vi "Show_Process_Steps.vi"(8 "error in (no error)":errorcluster, 10 "ProcessSettingIn":T8[](array[typedef]), 11 "ProcessSteps":refnum<vi>) -> (0 "error out":errorcluster)   [LabVIEW 2019]
uses:
  Controls/MaskParam_Type.ctl
  Controls/BinaryMonoParam_Type.ctl
  Controls/Process_Setting.ctl
  Controls/OperatorsParam_Type.ctl
  Controls/GrayMorphologyParam_Type.ctl
  Controls/FiltersParam_Type.ctl
  Controls/LookupTableParam.ctl
  Controls/ParticleFilterParam_Type.ctl
  Controls/ExtractPlanParam_Type.ctl
  Ctrl/VisionProcessName.ctl
panel:
  in  "ExtractPlanParam":T1={"Color Plane"=enum."Blue"}
  in  "ParticleFilterParam":T2={"Selection Values"=[{"Measurement Parameter"=16, "Range Lower Value"=0.0, "Range Upper Value"=0.0, "Range"=FALSE, "Measurement Type"=FALSE}], "Keep/Remove Particles (F)"=FALSE, "Reject Border? (F)"=FALSE, "Fill Holes? (F)"=FALSE, "Connectivity 4/8 (8)"=FALSE} {"Selection Values"."Measurement Parameter" items=["Center of Mass X", "Center of Mass Y", "First Pixel X", "First Pixel Y", "Bounding Rect Left", "Bounding Rect Top", "Bounding Rect Right", "Bounding Rect Bottom", "Max Feret Diameter Start X", "Max Feret Diameter Start Y", "Max Feret Diameter End X", "Max Feret Diameter End Y", "Max Horiz. Segment Length Left", "Max Horiz. Segment Length Right", "Max Horiz. Segment Length Row", "-", "Bounding Rect Width", "Bounding Rect Height", "Bounding Rect Diagonal", "Perimeter", "Convex Hull Perimeter", "Holes' Perimeter", "Max Feret Diameter", "Equivalent Ellipse Major Axis", "Equivalent Ellipse Minor Axis", "Equivalent Ellipse Minor Axis (Feret)", "Equivalent Rect Long Side", "Equivalent Rect Short Side", "Equivalent Rect Diagonal", "Equivalent Rect Short Side (Feret)", "Average Horiz. Segment Length", "Average Vert. Segment Length", "Hydraulic Radius", "Waddel Disk Diameter", "-", "Area", "Holes' Area", "Particle & Holes' Area", "Convex Hull Area", "Image Area", "-", "Number of Holes", "Number of Horiz. Segments", "Number of Vert. Segments", "-", "Orientation", "Max Feret Diameter Orientation", "-", "% Area/Image Area", "% Area/(Particle & Holes' Area)", "Ratio of Equivalent Ellipse Axes", "Ratio of Equivalent Rect Sides", "-", "Elongation Factor", "Compactness Factor", "Heywood Circularity Factor", "Type Factor", "-", "Sum X", "Sum Y", "Sum XX", "Sum XY", "Sum YY", "Sum XXX", "Sum XXY", "Sum XYY", "Sum YYY", "-", "Moment of Inertia XX", "Moment of Inertia XY", "Moment of Inertia YY", "Moment of Inertia XXX", "Moment of Inertia XXY", "Moment of Inertia XYY", "Moment of Inertia YYY", "Norm. Moment of Inertia XX", "Norm. Moment of Inertia XY", "Norm. Moment of Inertia YY", "Norm. Moment of Inertia XXX", "Norm. Moment of Inertia XXY", "Norm. Moment of Inertia XYY", "Norm. Moment of Inertia YYY", "Hu Moment 1", "Hu Moment 2", "Hu Moment 3", "Hu Moment 4", "Hu Moment 5", "Hu Moment 6", "Hu Moment 7"]; "Selection Values"."Range Lower Value" format="%.2f"; "Selection Values"."Range Upper Value" format="%.2f"}
  in  "LookupTableParam":T4
  in  "FiltersParam":T5={"Kernel"=[[1.0, 1.0, 1.0], [1.0, 1.0, 1.0], [1.0, 1.0, 1.0]], "Kernel Size"=0, "Filter Size X"=0, "Filter Size Y"=0, "Tolerance %"=0, "Divider"=0.0, "FilterFunction"=enum."Smoothing - Low Pass", "Sigma"=0.0, "LThres"=0.0, "HThresh"=0.0, "Windows Size"=0} {"Kernel Size" min=3 max=7 step=2}
  in  "GrayMorphologyParam":T6={"Operation"=enum."Gradient in", "Structuring Element"=[[1, 1, 1], [1, 1, 1], [1, 1, 1]], "Square/Hexa (Square)"=TRUE, "Number of iterations"=1}
  in  "OperatorsParam":T7
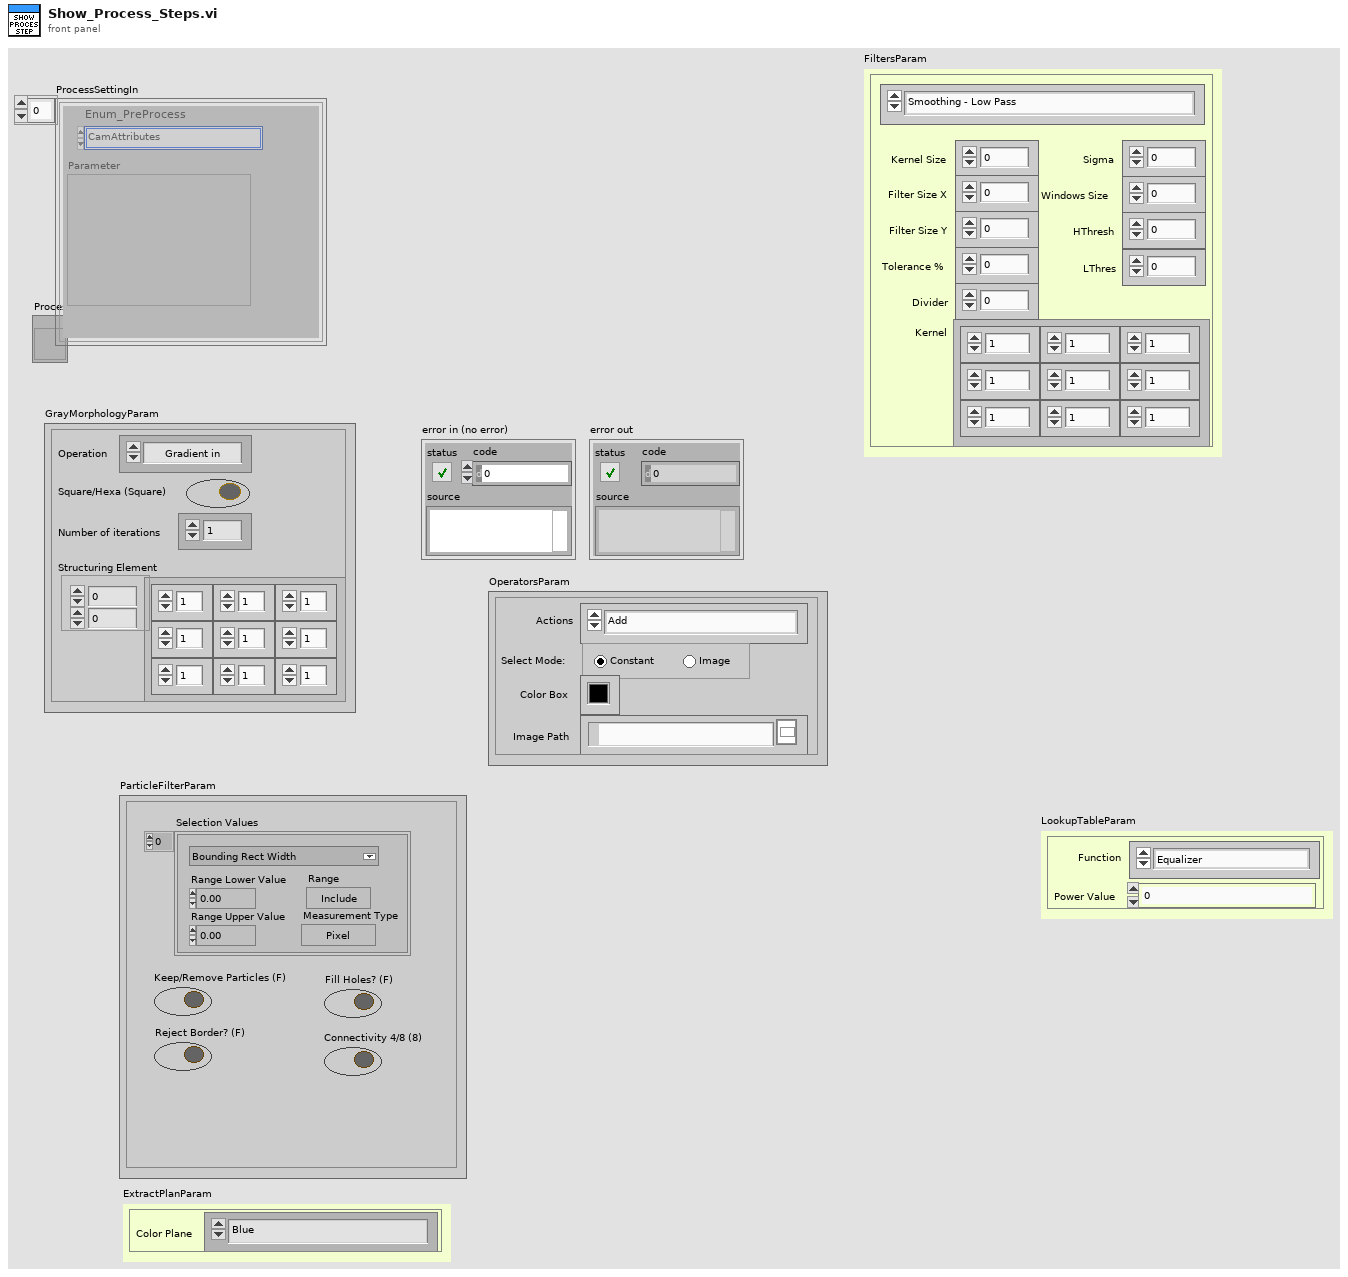
[diagram p1: front panel]
types:
  T1 = typedef "ExtractPlanParam_Type.ctl" = cluster{"Color Plane":enum16{"Red", "Green", "Blue", "Hue", "Saturation", "Luminance", "Value", "Intensity"}}
  T2 = typedef "ParticleFilterParam_Type.ctl" = cluster{"Selection Values":cluster{"Measurement Parameter":T3, "Range Lower Value":dbl, "Range Upper Value":dbl, "Range":bool, "Measurement Type":bool}[], "Keep/Remove Particles (F)":bool, "Reject Border? (F)":bool, "Fill Holes? (F)":bool, "Connectivity 4/8 (8)":bool}
  T3 = typedef "Particle Parameters" = i32
  T4 = typedef "LookupTableParam.ctl" = cluster{"Function":enum16{"Equalizer", "Reverse", "Logarithmic", "Exponential", "Square", "Square Root", "Power X", "Power 1/X"}, "Power Value":sgl}
  T5 = typedef "FiltersParam_Type.ctl" = cluster{"Kernel":sgl[][], "Kernel Size":i32, "Filter Size X":i32, "Filter Size Y":i32, "Tolerance %":i32, "Divider":sgl, "FilterFunction":enum16{"Smoothing - Low Pass", "Smoothing - Local Average", "Smoothing - Guassian", "Smoothing - Median", "------------------------------------", "Edge Detection - Laplacian", "Edge Detection - Diff", "Edge Detection - Prewitt", "Edge Detection - Sobel", "Edge Detection - Roberts", "Edge Detection - Canny", "Edge Detection - Gradient", "Edge Detection - Sigma", "----------------------------------------", "Convolution - Highlight Details", "Convolution - Custom"}, "Sigma":sgl, "LThres":sgl, "HThresh":sgl, "Windows Size":i32}
  T6 = typedef "GrayMorphologyParam_Type.ctl" = cluster{"Operation":enum32{"AutoM", "Close", "Dilate", "Erode", "Gradient", "Gradient in", "Gradient out", "HitMiss", "Open", "PClose", "POpen", "Thick", "Thin"}, "Structuring Element":i32[][], "Square/Hexa (Square)":bool, "Number of iterations":i32}
  T7 = typedef "OperatorsParam_Type.ctl" = cluster{"Actions":enum16{"Add", "Subtract", "Multiply", "Divide", "Multiply Divide", "Modulo", "Absolutio Difference", "---------------------------------", "And", "Not And", "Or", "Not Or", "Exclusive Or", "Not Exclusive Or", "Logical Difference", "----------------------------------", "Mask"}, "Select Mode:":enum32{"Constant", "Image"}, "Color Box":u32, "Image Path":path}
  T8 = typedef "Process_Setting.ctl" = cluster{"Enum_PreProcess":T9, "Parameter":string}
  T9 = typedef "VisionProcessName.ctl" = enum16{"*CamParameter*", "CamAttributes", "*Preprocess*", "CG_Brightness", "C_Plane Extraction", "C_Threshold", "G_Lookup Table", "G_Threshold"}
  T10 = typedef "MaskParam_Type.ctl" = cluster{"Function":enum16{"Inside", "Outside"}, "ROI List":i32, "ROI":cluster{"Global Rectangle":i32[], "Contours":cluster{"Contour Type":u32, "ROI Type":u32, "Points":i32[]}[]}[], "Creat ROI":bool, "Delete ROI":bool, "Enabled/Disabled":bool, "Color Box":u32, "Last Mouse Position":cluster{"X":i32, "Y":i32}}
  T11 = typedef "BinaryMonoParam_Type.ctl" = cluster{"Look For":enum16{"Bright Objects", "Dark Objects", "Gray Objects"}, "Threshold":cluster{dbl, dbl}}
  T12 = typedef "Process_Type.ctl" = enum16{"None", "ExtractPlane", "BinaryMono", "Operators", "GrayMorphology", "Filters", "Lookup Table", "Particle Filter", "Mask"}
  T13 = enum16{"Red", "Green", "Blue", "Hue", "Saturation", "Luminance", "Value", "Intensity"}
  T14 = enum16{"Add", "Subtract", "Multiply", "Divide", "Multiply Divide", "Modulo", "Absolutio Difference", "---------------------------------", "And", "Not And", "Or", "Not Or", "Exclusive Or", "Not Exclusive Or", "Logical Difference", "----------------------------------", "Mask"}
  T15 = enum32{"AutoM", "Close", "Dilate", "Erode", "Gradient", "Gradient in", "Gradient out", "HitMiss", "Open", "PClose", "POpen", "Thick", "Thin"}
  T16 = enum16{"Smoothing - Low Pass", "Smoothing - Local Average", "Smoothing - Guassian", "Smoothing - Median", "------------------------------------", "Edge Detection - Laplacian", "Edge Detection - Diff", "Edge Detection - Prewitt", "Edge Detection - Sobel", "Edge Detection - Roberts", "Edge Detection - Canny", "Edge Detection - Gradient", "Edge Detection - Sigma", "----------------------------------------", "Convolution - Highlight Details", "Convolution - Custom"}
  T17 = enum16{"Equalizer", "Reverse", "Logarithmic", "Exponential", "Square", "Square Root", "Power X", "Power 1/X"}
  T18 = cluster{"Measurement Parameter":T3, "Range Lower Value":dbl, "Range Upper Value":dbl, "Range":bool, "Measurement Type":bool}[]
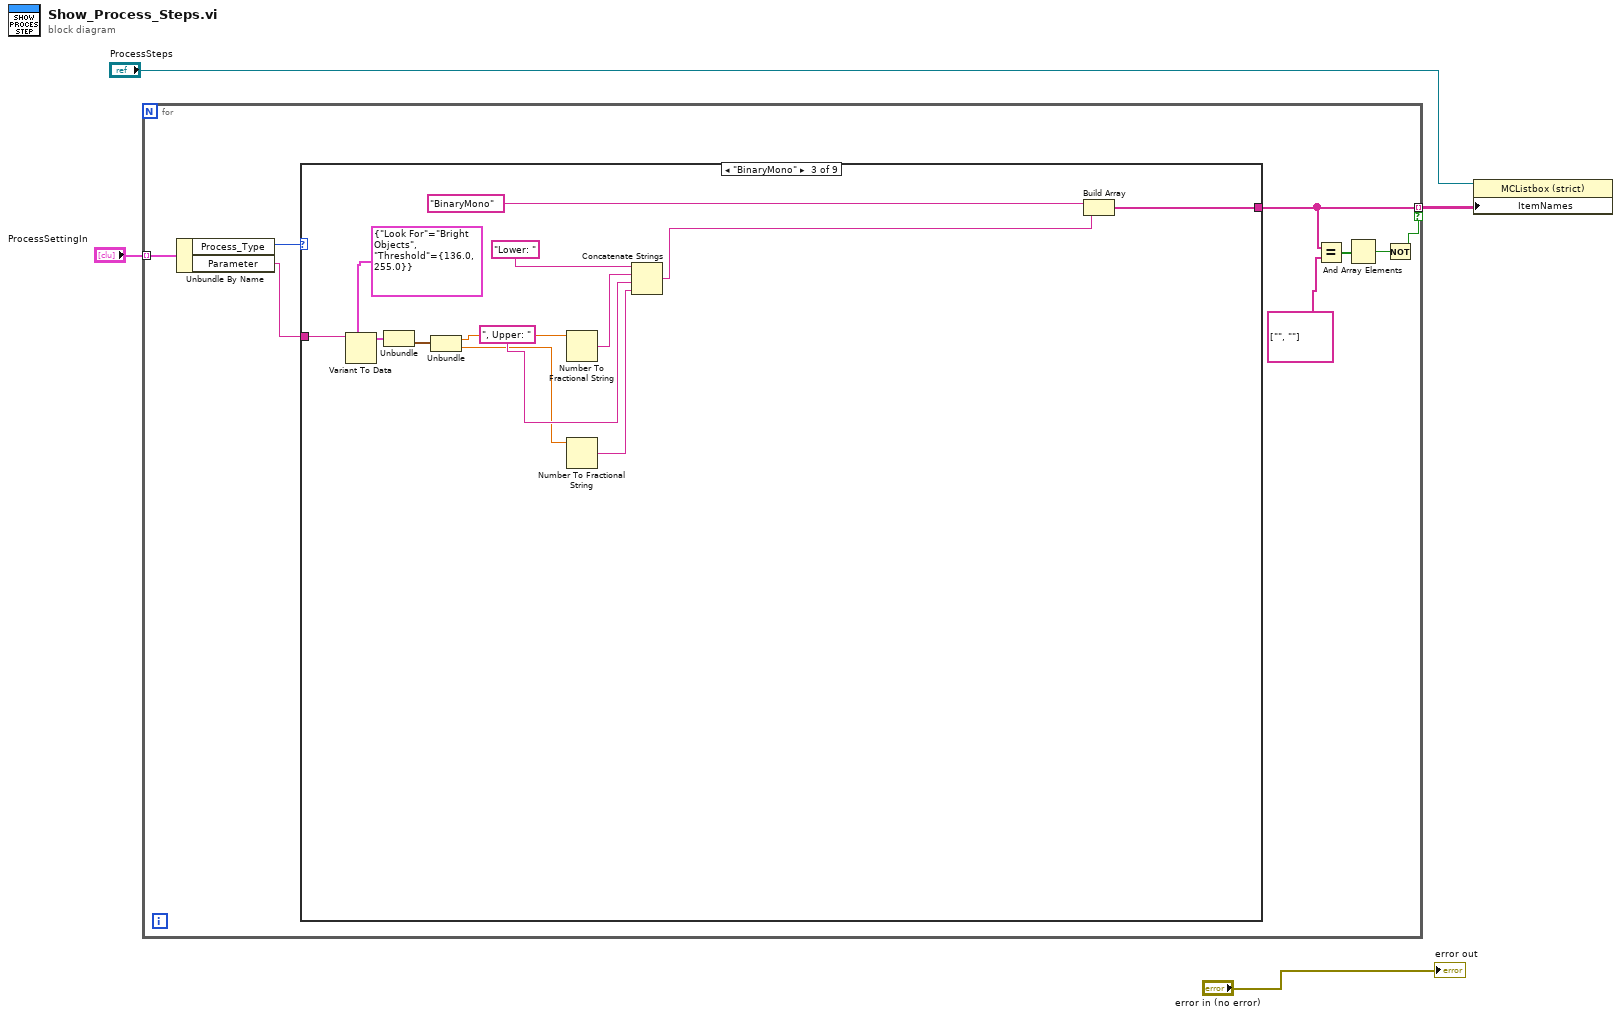
[diagram p0: block diagram]
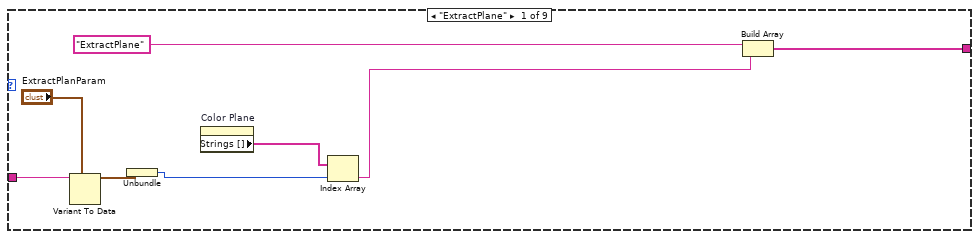
[diagram p2: hidden frame]
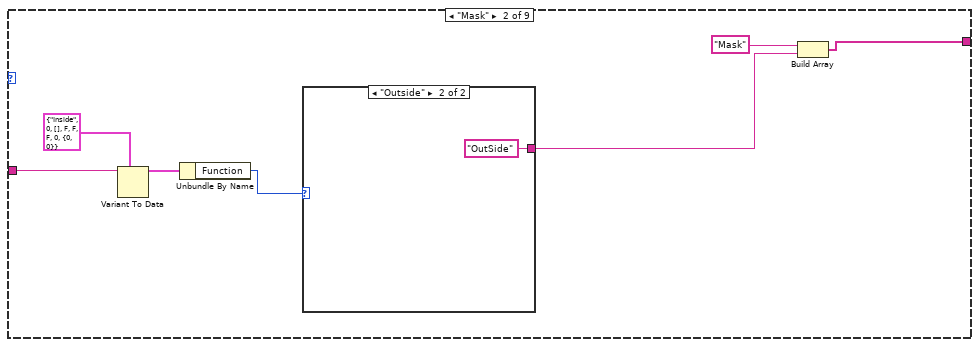
[diagram p3: hidden frame]
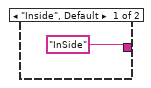
[diagram p4: hidden frame]
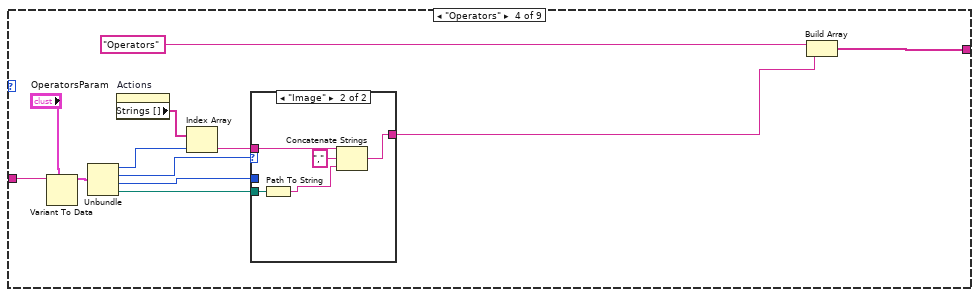
[diagram p5: hidden frame]
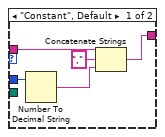
[diagram p6: hidden frame]
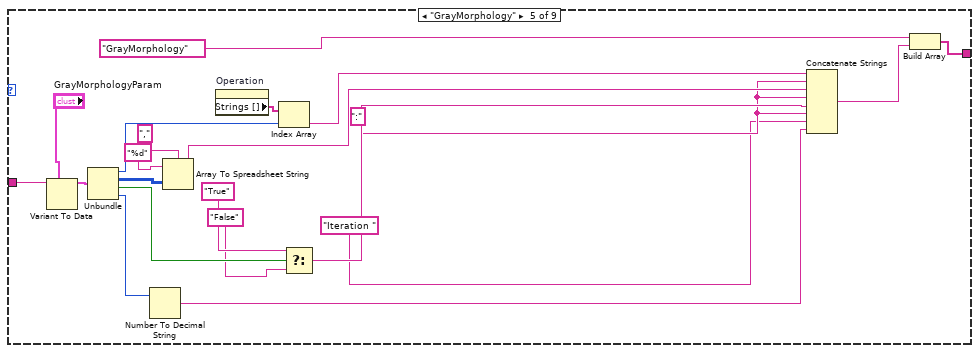
[diagram p7: hidden frame]
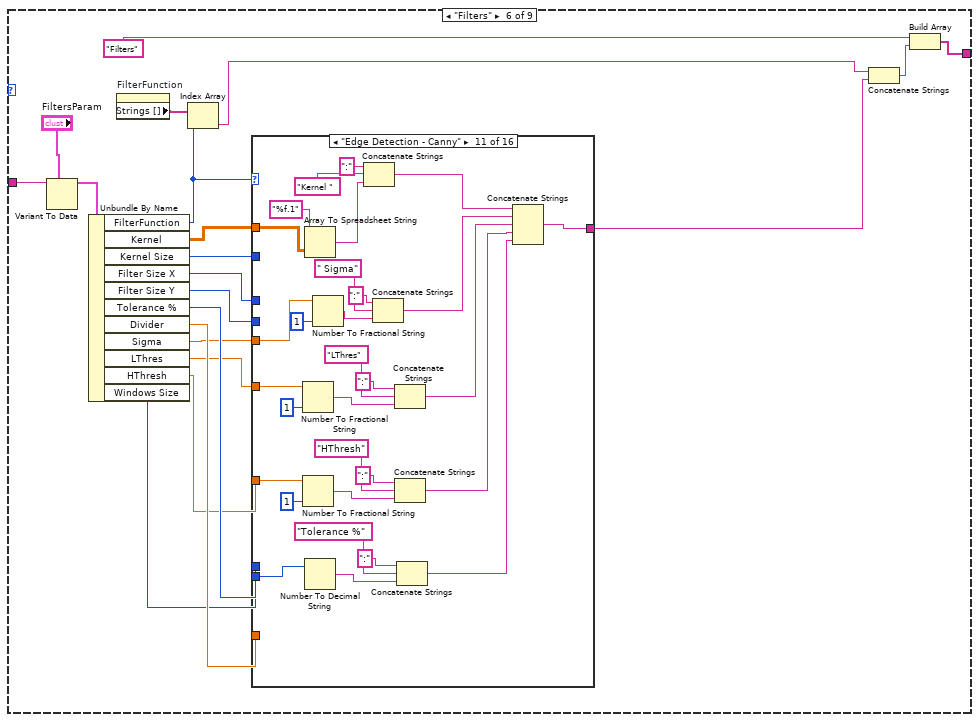
[diagram p8: hidden frame]
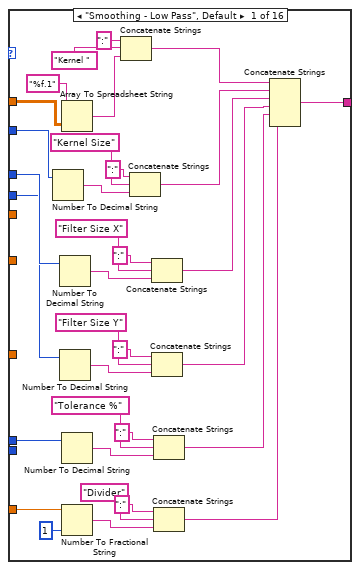
[diagram p9: hidden frame]
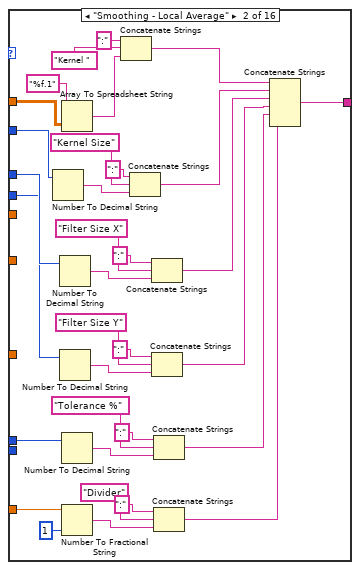
[diagram p10: hidden frame]
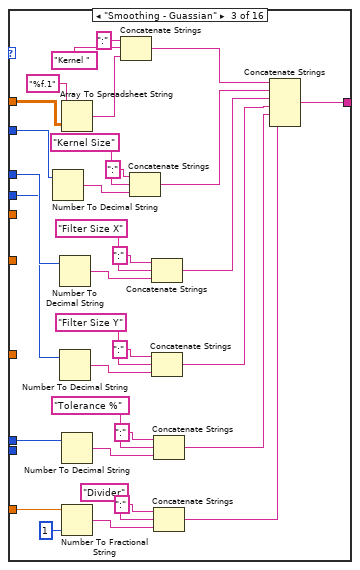
[diagram p11: hidden frame]
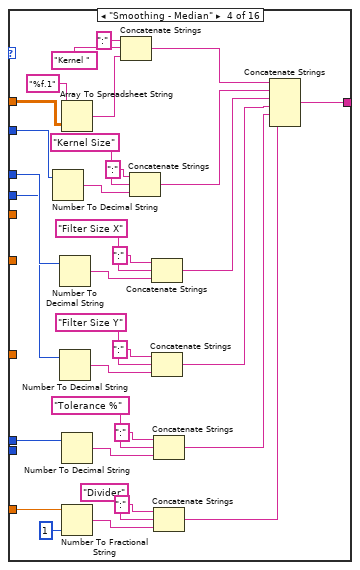
[diagram p12: hidden frame]
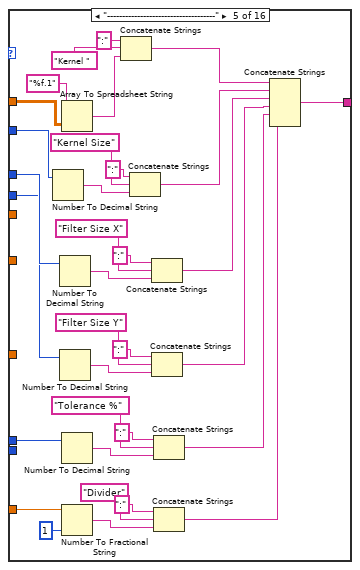
[diagram p13: hidden frame]
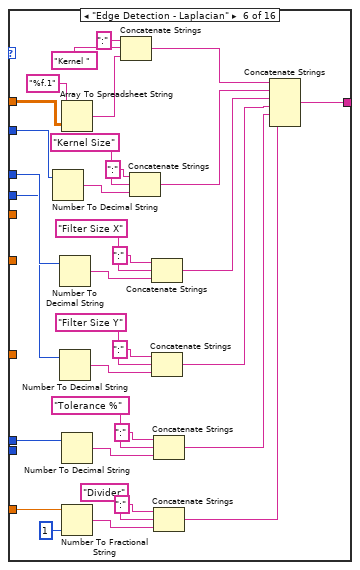
[diagram p14: hidden frame]
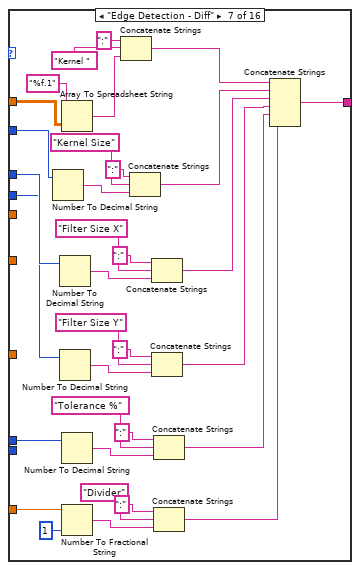
[diagram p15: hidden frame]
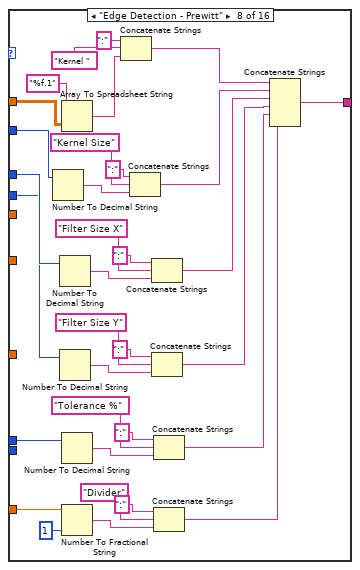
[diagram p16: hidden frame]
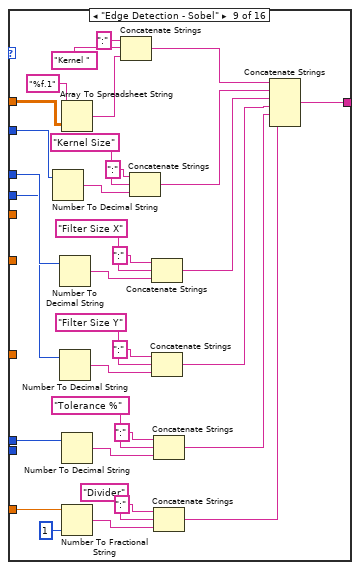
[diagram p17: hidden frame]
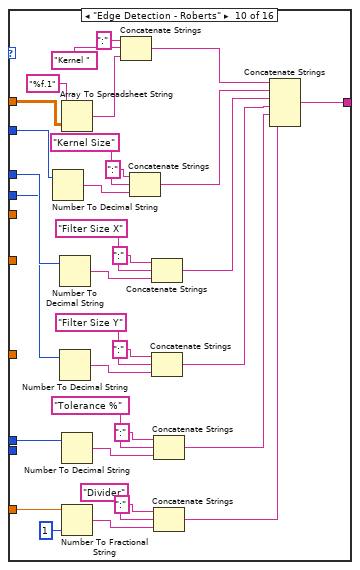
[diagram p18: hidden frame]
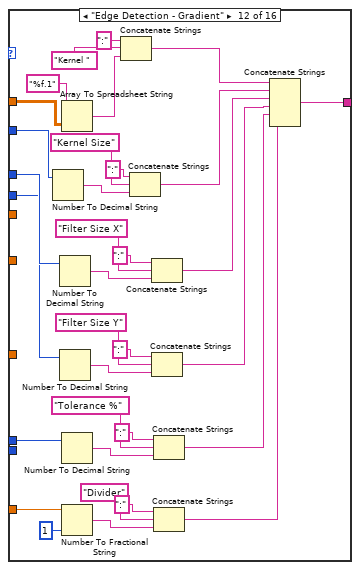
[diagram p19: hidden frame]
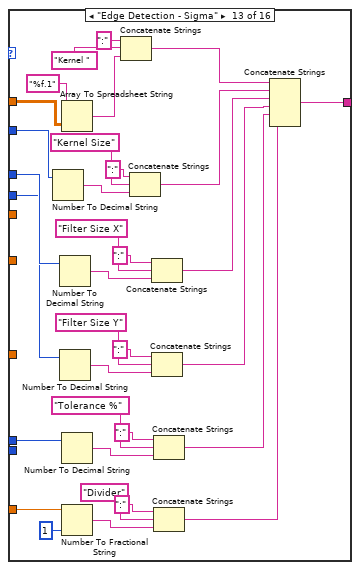
[diagram p20: hidden frame]
diagram:
  n1 = for {
    tunnel: "ProcessSettingIn" -> [w12] mode=indexing
    tunnel: [w9] -> w2 mode=indexing if=w5
    n2 = Unbundle By Name(w12) -> ("Process_Type"=w11:T12, "Parameter"=w10:string)
    n3 = case shown="\"BinaryMono\"" w11 {
      tunnel: w10 -> [w20 w25 w42 w54 w85 w105 w640 w696 _]
      tunnel: [w17 w27 w40 w43 w67 w103 w631 w693 _] -> w9
      frame "ExtractPlane" {
        n4 = Variant To Data(type="ExtractPlanParam", Variant=w20) -> (data=w16:T1)  [unwired: 1 in, 1 out]
        n5 = Unbundle(w16) -> ("Color Plane"=w15:T13)
        n6 = property on="Color Plane" class="Enum (strict)"() -> ("Strings []"=w14:string[])  [unwired: 2 in, 2 out]
        n7 = Index Array(array=w14, index=w15) -> (element=w18:string)
        n8 = Build Array("ExtractPlane", w18) -> (w17:string[])
      }
      frame "Mask" {
        n9 = Variant To Data(type=T10 {"Function"=enum."Inside", "ROI List"=0, "ROI"=[], "Creat ROI"=FALSE, "Delete ROI"=FALSE, "Enabled/Disabled"=FALSE, "Color Box"=0, "Last Mouse Position"={"X"=0, "Y"=0}} ("MaskParam"), Variant=w25) -> (data=w23:T10)  [unwired: 1 in, 1 out]
        n10 = Unbundle By Name(w23) -> ("Function"=w22:enum16{"Inside", "Outside"})
        n11 = case shown="\"Outside\"" w22 {
          tunnel: ["InSide" "OutSide"] -> w21
          frame "Inside", Default {
          }
          frame "Outside" {
          }
        }
        n12 = Build Array("Mask", w21) -> (w27:string[])
      }
      frame "BinaryMono" {
        n13 = Variant To Data(type=T11 {"Look For"=enum."Bright Objects", "Threshold"={136.0, 255.0}} ("BinaryMonoParam"), Variant=w42) -> (data=w34:T11)  [unwired: 1 in, 1 out]
        n14 = Unbundle(w34) -> ("Threshold"=w33:cluster{dbl, dbl})  [unwired: 1 out]
        n15 = Unbundle(w33) -> (w31:dbl, w32:dbl)
        n16 = Number To Fractional String(number=w31) -> (F-format string=w37:string)  [unwired: 3 in]
        n17 = Number To Fractional String(number=w32) -> (F-format string=w35:string)  [unwired: 3 in]
        n18 = Concatenate Strings("Lower: " ("string"), w37, ", Upper: " ("string"), w35) -> (w38:string)
        n19 = Build Array("BinaryMono", w38) -> (w40:string[])
      }
      frame "Operators" {
        n20 = Variant To Data(type="OperatorsParam", Variant=w54) -> (data=w52:T7)  [unwired: 1 in, 1 out]
        n21 = Unbundle(w52) -> ("Actions"=w49:T14, "Select Mode:"=w51:enum32{"Constant", "Image"}, "Color Box"=w47:u32, "Image Path"=w44:path)
        n22 = property on="Actions" class="Enum (strict)"() -> ("Strings []"=w50:string[])  [unwired: 2 in, 2 out]
        n23 = Index Array(array=w50, index=w49) -> (element=w48:string)
        n24 = case shown="\"Image\"" w51 {
          tunnel: w48 -> [w58 w64]
          tunnel: w47 -> [w59 _]
          tunnel: [w55 w62] -> w45
          tunnel: w44 -> [_ w61]
          frame "Constant", Default {
            n25 = Number To Decimal String(number=w59) -> (decimal integer string=w56:string)  [unwired: 1 in]
            n26 = Concatenate Strings(w58, "," ("string"), w56) -> (w55:string)
          }
          frame "Image" {
            n27 = Path To String(path=w61) -> (string=w60:string)
            n28 = Concatenate Strings(w64, "," ("string"), w60) -> (w62:string)
          }
        }
        n29 = Build Array("Operators", w45) -> (w43:string[])
      }
      frame "GrayMorphology" {
        w71 = ":" ("element")
        n30 = Variant To Data(type="GrayMorphologyParam", Variant=w85) -> (data=w84:T6)  [unwired: 1 in, 1 out]
        n31 = Unbundle(w84) -> ("Operation"=w81:T15, "Structuring Element"=w80:i32[][], "Square/Hexa (Square)"=w75:bool, "Number of iterations"=w70:i32)
        n32 = Number To Decimal String(number=w70) -> (decimal integer string=w66:string)  [unwired: 1 in]
        n33 = Array To Spreadsheet String(delimiter (Tab)=",", array=w80, 3:"%d" ("format string")) -> (spreadsheet string=w76:string)
        n34 = property on="Operation" class="Enum (strict)"() -> ("Strings []"=w82:string[])  [unwired: 2 in, 2 out]
        n35 = Index Array(array=w82, index=w81) -> (element=w77:string)
        n36 = Select(t="True" ("delimiter (Tab)"), s=w75, f="False" ("delimiter (Tab)")) -> (s? t:f=w72:string)
        n37 = Concatenate Strings(w77, w71, w76, w71, w72, w71, "Iteration " ("string"), w66) -> (w69:string)
        n38 = Build Array("GrayMorphology", w69) -> (w67:string[])
      }
      frame "Filters" {
        n39 = Variant To Data(type="FiltersParam", Variant=w105) -> (data=w100:T5)  [unwired: 1 in, 1 out]
        n40 = Unbundle By Name(w100) -> ("FilterFunction"=w99:T16, "Kernel"=w98:sgl[][], "Kernel Size"=w96:i32, "Filter Size X"=w95:i32, "Filter Size Y"=w94:i32, "Tolerance %"=w93:i32, "Divider"=w92:sgl, "Sigma"=w89:sgl, "LThres"=w88:sgl, "HThresh"=w87:sgl, "Windows Size"=w86:i32)
        n41 = property on="FilterFunction" class="Enum (strict)"() -> ("Strings []"=w101:string[])  [unwired: 2 in, 2 out]
        n42 = Index Array(array=w101, index=w99) -> (element=w97:string)
        n43 = case shown="\"Edge Detection - Canny\"" w99 {
          tunnel: w98 -> [w136 w169 w202 w235 w268 w301 w334 w367 w400 w433 w463 w496 w529 w562 w595 w628]
          tunnel: w96 -> [w133 w166 w199 w232 w265 w298 w331 w364 w397 w430 _ w493 w526 w559 w592 w625]
          tunnel: w95 -> [w126 w159 w192 w225 w258 w291 w324 w357 w390 w423 _ w486 w519 w552 w585 w618]
          tunnel: w94 -> [w122 w155 w188 w221 w254 w287 w320 w353 w386 w419 _ w482 w515 w548 w581 w614]
          tunnel: w93 -> [w118 w151 w184 w217 w250 w283 w316 w349 w382 w415 _ w478 w511 w544 w577 w610]
          tunnel: w92 -> [w113 w146 w179 w212 w245 w278 w311 w344 w377 w410 _ w473 w506 w539 w572 w605]
          tunnel: [w106 w139 w172 w205 w238 w271 w304 w337 w370 w403 w443 w466 w499 w532 w565 w598] -> w91
          tunnel: w89 -> [_ _ _ _ _ _ _ _ _ _ w442 _ _ _ _ _]
          tunnel: w88 -> [_ _ _ _ _ _ _ _ _ _ w440 _ _ _ _ _]
          tunnel: w87 -> [_ _ _ _ _ _ _ _ _ _ w438 _ _ _ _ _]
          tunnel: w86 -> [_ _ _ _ _ _ _ _ _ _ w436 _ _ _ _ _]
          frame "Smoothing - Low Pass", Default {
            n44 = Number To Decimal String(number=w133) -> (decimal integer string=w131:string)  [unwired: 1 in]
            n45 = Number To Decimal String(number=w126) -> (decimal integer string=w128:string)  [unwired: 1 in]
            n46 = Number To Decimal String(number=w122) -> (decimal integer string=w124:string)  [unwired: 1 in]
            n47 = Array To Spreadsheet String(array=w136, 3:"%f.1" ("format string")) -> (spreadsheet string=w134:string)  [unwired: 1 in]
            n48 = Number To Decimal String(number=w118) -> (decimal integer string=w120:string)  [unwired: 1 in]
            n49 = Number To Fractional String(number=w113, precision (6)=i16 1) -> (F-format string=w116:string)  [unwired: 2 in]
            n50 = Concatenate Strings(":" ("string"), "Kernel " ("string"), w134) -> (w112:string)
            n51 = Concatenate Strings(":" ("string"), "Kernel Size" ("string"), w131) -> (w111:string)
            n52 = Concatenate Strings(":" ("string"), "Filter Size X" ("string"), w128) -> (w110:string)
            n53 = Concatenate Strings(":" ("string"), "Filter Size Y" ("string"), w124) -> (w109:string)
            n54 = Concatenate Strings(":" ("string"), "Tolerance %" ("string"), w120) -> (w108:string)
            n55 = Concatenate Strings(":" ("string"), "Divider" ("string"), w116) -> (w107:string)
            n56 = Concatenate Strings(w112, w111, w110, w109, w108, w107) -> (w106:string)
          }
          frame "Smoothing - Local Average" {
            n57 = Number To Decimal String(number=w166) -> (decimal integer string=w164:string)  [unwired: 1 in]
            n58 = Number To Decimal String(number=w159) -> (decimal integer string=w161:string)  [unwired: 1 in]
            n59 = Number To Decimal String(number=w155) -> (decimal integer string=w157:string)  [unwired: 1 in]
            n60 = Array To Spreadsheet String(array=w169, 3:"%f.1" ("format string")) -> (spreadsheet string=w167:string)  [unwired: 1 in]
            n61 = Number To Decimal String(number=w151) -> (decimal integer string=w153:string)  [unwired: 1 in]
            n62 = Number To Fractional String(number=w146, precision (6)=i16 1) -> (F-format string=w149:string)  [unwired: 2 in]
            n63 = Concatenate Strings(":" ("string"), "Kernel " ("string"), w167) -> (w145:string)
            n64 = Concatenate Strings(":" ("string"), "Kernel Size" ("string"), w164) -> (w144:string)
            n65 = Concatenate Strings(":" ("string"), "Filter Size X" ("string"), w161) -> (w143:string)
            n66 = Concatenate Strings(":" ("string"), "Filter Size Y" ("string"), w157) -> (w142:string)
            n67 = Concatenate Strings(":" ("string"), "Tolerance %" ("string"), w153) -> (w141:string)
            n68 = Concatenate Strings(":" ("string"), "Divider" ("string"), w149) -> (w140:string)
            n69 = Concatenate Strings(w145, w144, w143, w142, w141, w140) -> (w139:string)
          }
          frame "Smoothing - Guassian" {
            n70 = Number To Decimal String(number=w199) -> (decimal integer string=w197:string)  [unwired: 1 in]
            n71 = Number To Decimal String(number=w192) -> (decimal integer string=w194:string)  [unwired: 1 in]
            n72 = Number To Decimal String(number=w188) -> (decimal integer string=w190:string)  [unwired: 1 in]
            n73 = Array To Spreadsheet String(array=w202, 3:"%f.1" ("format string")) -> (spreadsheet string=w200:string)  [unwired: 1 in]
            n74 = Number To Decimal String(number=w184) -> (decimal integer string=w186:string)  [unwired: 1 in]
            n75 = Number To Fractional String(number=w179, precision (6)=i16 1) -> (F-format string=w182:string)  [unwired: 2 in]
            n76 = Concatenate Strings(":" ("string"), "Kernel " ("string"), w200) -> (w178:string)
            n77 = Concatenate Strings(":" ("string"), "Kernel Size" ("string"), w197) -> (w177:string)
            n78 = Concatenate Strings(":" ("string"), "Filter Size X" ("string"), w194) -> (w176:string)
            n79 = Concatenate Strings(":" ("string"), "Filter Size Y" ("string"), w190) -> (w175:string)
            n80 = Concatenate Strings(":" ("string"), "Tolerance %" ("string"), w186) -> (w174:string)
            n81 = Concatenate Strings(":" ("string"), "Divider" ("string"), w182) -> (w173:string)
            n82 = Concatenate Strings(w178, w177, w176, w175, w174, w173) -> (w172:string)
          }
          frame "Smoothing - Median" {
            n83 = Number To Decimal String(number=w232) -> (decimal integer string=w230:string)  [unwired: 1 in]
            n84 = Number To Decimal String(number=w225) -> (decimal integer string=w227:string)  [unwired: 1 in]
            n85 = Number To Decimal String(number=w221) -> (decimal integer string=w223:string)  [unwired: 1 in]
            n86 = Array To Spreadsheet String(array=w235, 3:"%f.1" ("format string")) -> (spreadsheet string=w233:string)  [unwired: 1 in]
            n87 = Number To Decimal String(number=w217) -> (decimal integer string=w219:string)  [unwired: 1 in]
            n88 = Number To Fractional String(number=w212, precision (6)=i16 1) -> (F-format string=w215:string)  [unwired: 2 in]
            n89 = Concatenate Strings(":" ("string"), "Kernel " ("string"), w233) -> (w211:string)
            n90 = Concatenate Strings(":" ("string"), "Kernel Size" ("string"), w230) -> (w210:string)
            n91 = Concatenate Strings(":" ("string"), "Filter Size X" ("string"), w227) -> (w209:string)
            n92 = Concatenate Strings(":" ("string"), "Filter Size Y" ("string"), w223) -> (w208:string)
            n93 = Concatenate Strings(":" ("string"), "Tolerance %" ("string"), w219) -> (w207:string)
            n94 = Concatenate Strings(":" ("string"), "Divider" ("string"), w215) -> (w206:string)
            n95 = Concatenate Strings(w211, w210, w209, w208, w207, w206) -> (w205:string)
          }
          frame "------------------------------------" {
            n96 = Number To Decimal String(number=w265) -> (decimal integer string=w263:string)  [unwired: 1 in]
            n97 = Number To Decimal String(number=w258) -> (decimal integer string=w260:string)  [unwired: 1 in]
            n98 = Number To Decimal String(number=w254) -> (decimal integer string=w256:string)  [unwired: 1 in]
            n99 = Array To Spreadsheet String(array=w268, 3:"%f.1" ("format string")) -> (spreadsheet string=w266:string)  [unwired: 1 in]
            n100 = Number To Decimal String(number=w250) -> (decimal integer string=w252:string)  [unwired: 1 in]
            n101 = Number To Fractional String(number=w245, precision (6)=i16 1) -> (F-format string=w248:string)  [unwired: 2 in]
            n102 = Concatenate Strings(":" ("string"), "Kernel " ("string"), w266) -> (w244:string)
            n103 = Concatenate Strings(":" ("string"), "Kernel Size" ("string"), w263) -> (w243:string)
            n104 = Concatenate Strings(":" ("string"), "Filter Size X" ("string"), w260) -> (w242:string)
            n105 = Concatenate Strings(":" ("string"), "Filter Size Y" ("string"), w256) -> (w241:string)
            n106 = Concatenate Strings(":" ("string"), "Tolerance %" ("string"), w252) -> (w240:string)
            n107 = Concatenate Strings(":" ("string"), "Divider" ("string"), w248) -> (w239:string)
            n108 = Concatenate Strings(w244, w243, w242, w241, w240, w239) -> (w238:string)
          }
          frame "Edge Detection - Laplacian" {
            n109 = Number To Decimal String(number=w298) -> (decimal integer string=w296:string)  [unwired: 1 in]
            n110 = Number To Decimal String(number=w291) -> (decimal integer string=w293:string)  [unwired: 1 in]
            n111 = Number To Decimal String(number=w287) -> (decimal integer string=w289:string)  [unwired: 1 in]
            n112 = Array To Spreadsheet String(array=w301, 3:"%f.1" ("format string")) -> (spreadsheet string=w299:string)  [unwired: 1 in]
            n113 = Number To Decimal String(number=w283) -> (decimal integer string=w285:string)  [unwired: 1 in]
            n114 = Number To Fractional String(number=w278, precision (6)=i16 1) -> (F-format string=w281:string)  [unwired: 2 in]
            n115 = Concatenate Strings(":" ("string"), "Kernel " ("string"), w299) -> (w277:string)
            n116 = Concatenate Strings(":" ("string"), "Kernel Size" ("string"), w296) -> (w276:string)
            n117 = Concatenate Strings(":" ("string"), "Filter Size X" ("string"), w293) -> (w275:string)
            n118 = Concatenate Strings(":" ("string"), "Filter Size Y" ("string"), w289) -> (w274:string)
            n119 = Concatenate Strings(":" ("string"), "Tolerance %" ("string"), w285) -> (w273:string)
            n120 = Concatenate Strings(":" ("string"), "Divider" ("string"), w281) -> (w272:string)
            n121 = Concatenate Strings(w277, w276, w275, w274, w273, w272) -> (w271:string)
          }
          frame "Edge Detection - Diff" {
            n122 = Number To Decimal String(number=w331) -> (decimal integer string=w329:string)  [unwired: 1 in]
            n123 = Number To Decimal String(number=w324) -> (decimal integer string=w326:string)  [unwired: 1 in]
            n124 = Number To Decimal String(number=w320) -> (decimal integer string=w322:string)  [unwired: 1 in]
            n125 = Array To Spreadsheet String(array=w334, 3:"%f.1" ("format string")) -> (spreadsheet string=w332:string)  [unwired: 1 in]
            n126 = Number To Decimal String(number=w316) -> (decimal integer string=w318:string)  [unwired: 1 in]
            n127 = Number To Fractional String(number=w311, precision (6)=i16 1) -> (F-format string=w314:string)  [unwired: 2 in]
            n128 = Concatenate Strings(":" ("string"), "Kernel " ("string"), w332) -> (w310:string)
            n129 = Concatenate Strings(":" ("string"), "Kernel Size" ("string"), w329) -> (w309:string)
            n130 = Concatenate Strings(":" ("string"), "Filter Size X" ("string"), w326) -> (w308:string)
            n131 = Concatenate Strings(":" ("string"), "Filter Size Y" ("string"), w322) -> (w307:string)
            n132 = Concatenate Strings(":" ("string"), "Tolerance %" ("string"), w318) -> (w306:string)
            n133 = Concatenate Strings(":" ("string"), "Divider" ("string"), w314) -> (w305:string)
            n134 = Concatenate Strings(w310, w309, w308, w307, w306, w305) -> (w304:string)
          }
          frame "Edge Detection - Prewitt" {
            n135 = Number To Decimal String(number=w364) -> (decimal integer string=w362:string)  [unwired: 1 in]
            n136 = Number To Decimal String(number=w357) -> (decimal integer string=w359:string)  [unwired: 1 in]
            n137 = Number To Decimal String(number=w353) -> (decimal integer string=w355:string)  [unwired: 1 in]
            n138 = Array To Spreadsheet String(array=w367, 3:"%f.1" ("format string")) -> (spreadsheet string=w365:string)  [unwired: 1 in]
            n139 = Number To Decimal String(number=w349) -> (decimal integer string=w351:string)  [unwired: 1 in]
            n140 = Number To Fractional String(number=w344, precision (6)=i16 1) -> (F-format string=w347:string)  [unwired: 2 in]
            n141 = Concatenate Strings(":" ("string"), "Kernel " ("string"), w365) -> (w343:string)
            n142 = Concatenate Strings(":" ("string"), "Kernel Size" ("string"), w362) -> (w342:string)
            n143 = Concatenate Strings(":" ("string"), "Filter Size X" ("string"), w359) -> (w341:string)
            n144 = Concatenate Strings(":" ("string"), "Filter Size Y" ("string"), w355) -> (w340:string)
            n145 = Concatenate Strings(":" ("string"), "Tolerance %" ("string"), w351) -> (w339:string)
            n146 = Concatenate Strings(":" ("string"), "Divider" ("string"), w347) -> (w338:string)
            n147 = Concatenate Strings(w343, w342, w341, w340, w339, w338) -> (w337:string)
          }
          frame "Edge Detection - Sobel" {
            n148 = Number To Decimal String(number=w397) -> (decimal integer string=w395:string)  [unwired: 1 in]
            n149 = Number To Decimal String(number=w390) -> (decimal integer string=w392:string)  [unwired: 1 in]
            n150 = Number To Decimal String(number=w386) -> (decimal integer string=w388:string)  [unwired: 1 in]
            n151 = Array To Spreadsheet String(array=w400, 3:"%f.1" ("format string")) -> (spreadsheet string=w398:string)  [unwired: 1 in]
            n152 = Number To Decimal String(number=w382) -> (decimal integer string=w384:string)  [unwired: 1 in]
            n153 = Number To Fractional String(number=w377, precision (6)=i16 1) -> (F-format string=w380:string)  [unwired: 2 in]
            n154 = Concatenate Strings(":" ("string"), "Kernel " ("string"), w398) -> (w376:string)
            n155 = Concatenate Strings(":" ("string"), "Kernel Size" ("string"), w395) -> (w375:string)
            n156 = Concatenate Strings(":" ("string"), "Filter Size X" ("string"), w392) -> (w374:string)
            n157 = Concatenate Strings(":" ("string"), "Filter Size Y" ("string"), w388) -> (w373:string)
            n158 = Concatenate Strings(":" ("string"), "Tolerance %" ("string"), w384) -> (w372:string)
            n159 = Concatenate Strings(":" ("string"), "Divider" ("string"), w380) -> (w371:string)
            n160 = Concatenate Strings(w376, w375, w374, w373, w372, w371) -> (w370:string)
          }
          frame "Edge Detection - Roberts" {
            n161 = Number To Decimal String(number=w430) -> (decimal integer string=w428:string)  [unwired: 1 in]
            n162 = Number To Decimal String(number=w423) -> (decimal integer string=w425:string)  [unwired: 1 in]
            n163 = Number To Decimal String(number=w419) -> (decimal integer string=w421:string)  [unwired: 1 in]
            n164 = Array To Spreadsheet String(array=w433, 3:"%f.1" ("format string")) -> (spreadsheet string=w431:string)  [unwired: 1 in]
            n165 = Number To Decimal String(number=w415) -> (decimal integer string=w417:string)  [unwired: 1 in]
            n166 = Number To Fractional String(number=w410, precision (6)=i16 1) -> (F-format string=w413:string)  [unwired: 2 in]
            n167 = Concatenate Strings(":" ("string"), "Kernel " ("string"), w431) -> (w409:string)
            n168 = Concatenate Strings(":" ("string"), "Kernel Size" ("string"), w428) -> (w408:string)
            n169 = Concatenate Strings(":" ("string"), "Filter Size X" ("string"), w425) -> (w407:string)
            n170 = Concatenate Strings(":" ("string"), "Filter Size Y" ("string"), w421) -> (w406:string)
            n171 = Concatenate Strings(":" ("string"), "Tolerance %" ("string"), w417) -> (w405:string)
            n172 = Concatenate Strings(":" ("string"), "Divider" ("string"), w413) -> (w404:string)
            n173 = Concatenate Strings(w409, w408, w407, w406, w405, w404) -> (w403:string)
          }
          frame "Edge Detection - Canny" {
            n174 = Number To Fractional String(number=w440, precision (6)=i16 1) -> (F-format string=w456:string)  [unwired: 2 in]
            n175 = Number To Fractional String(number=w438, precision (6)=i16 1) -> (F-format string=w453:string)  [unwired: 2 in]
            n176 = Array To Spreadsheet String(array=w463, 3:"%f.1" ("format string")) -> (spreadsheet string=w461:string)  [unwired: 1 in]
            n177 = Number To Decimal String(number=w436) -> (decimal integer string=w450:string)  [unwired: 1 in]
            n178 = Number To Fractional String(number=w442, precision (6)=i16 1) -> (F-format string=w459:string)  [unwired: 2 in]
            n179 = Concatenate Strings(":" ("string"), "Kernel " ("string"), w461) -> (w448:string)
            n180 = Concatenate Strings(":" ("string"), " Sigma" ("string"), w459) -> (w447:string)
            n181 = Concatenate Strings(":" ("string"), "LThres" ("string"), w456) -> (w446:string)
            n182 = Concatenate Strings(":" ("string"), "HThresh" ("string"), w453) -> (w445:string)
            n183 = Concatenate Strings(":" ("string"), "Tolerance %" ("string"), w450) -> (w444:string)
            n184 = Concatenate Strings(w448, w447, w446, w445, w444) -> (w443:string)
          }
          frame "Edge Detection - Gradient" {
            n185 = Number To Decimal String(number=w493) -> (decimal integer string=w491:string)  [unwired: 1 in]
            n186 = Number To Decimal String(number=w486) -> (decimal integer string=w488:string)  [unwired: 1 in]
            n187 = Number To Decimal String(number=w482) -> (decimal integer string=w484:string)  [unwired: 1 in]
            n188 = Array To Spreadsheet String(array=w496, 3:"%f.1" ("format string")) -> (spreadsheet string=w494:string)  [unwired: 1 in]
            n189 = Number To Decimal String(number=w478) -> (decimal integer string=w480:string)  [unwired: 1 in]
            n190 = Number To Fractional String(number=w473, precision (6)=i16 1) -> (F-format string=w476:string)  [unwired: 2 in]
            n191 = Concatenate Strings(":" ("string"), "Kernel " ("string"), w494) -> (w472:string)
            n192 = Concatenate Strings(":" ("string"), "Kernel Size" ("string"), w491) -> (w471:string)
            n193 = Concatenate Strings(":" ("string"), "Filter Size X" ("string"), w488) -> (w470:string)
            n194 = Concatenate Strings(":" ("string"), "Filter Size Y" ("string"), w484) -> (w469:string)
            n195 = Concatenate Strings(":" ("string"), "Tolerance %" ("string"), w480) -> (w468:string)
            n196 = Concatenate Strings(":" ("string"), "Divider" ("string"), w476) -> (w467:string)
            n197 = Concatenate Strings(w472, w471, w470, w469, w468, w467) -> (w466:string)
          }
          frame "Edge Detection - Sigma" {
            n198 = Number To Decimal String(number=w526) -> (decimal integer string=w524:string)  [unwired: 1 in]
            n199 = Number To Decimal String(number=w519) -> (decimal integer string=w521:string)  [unwired: 1 in]
            n200 = Number To Decimal String(number=w515) -> (decimal integer string=w517:string)  [unwired: 1 in]
            n201 = Array To Spreadsheet String(array=w529, 3:"%f.1" ("format string")) -> (spreadsheet string=w527:string)  [unwired: 1 in]
            n202 = Number To Decimal String(number=w511) -> (decimal integer string=w513:string)  [unwired: 1 in]
            n203 = Number To Fractional String(number=w506, precision (6)=i16 1) -> (F-format string=w509:string)  [unwired: 2 in]
            n204 = Concatenate Strings(":" ("string"), "Kernel " ("string"), w527) -> (w505:string)
            n205 = Concatenate Strings(":" ("string"), "Kernel Size" ("string"), w524) -> (w504:string)
            n206 = Concatenate Strings(":" ("string"), "Filter Size X" ("string"), w521) -> (w503:string)
            n207 = Concatenate Strings(":" ("string"), "Filter Size Y" ("string"), w517) -> (w502:string)
            n208 = Concatenate Strings(":" ("string"), "Tolerance %" ("string"), w513) -> (w501:string)
            n209 = Concatenate Strings(":" ("string"), "Divider" ("string"), w509) -> (w500:string)
            n210 = Concatenate Strings(w505, w504, w503, w502, w501, w500) -> (w499:string)
          }
          frame "----------------------------------------" {
            n211 = Number To Decimal String(number=w559) -> (decimal integer string=w557:string)  [unwired: 1 in]
            n212 = Number To Decimal String(number=w552) -> (decimal integer string=w554:string)  [unwired: 1 in]
            n213 = Number To Decimal String(number=w548) -> (decimal integer string=w550:string)  [unwired: 1 in]
            n214 = Array To Spreadsheet String(array=w562, 3:"%f.1" ("format string")) -> (spreadsheet string=w560:string)  [unwired: 1 in]
            n215 = Number To Decimal String(number=w544) -> (decimal integer string=w546:string)  [unwired: 1 in]
            n216 = Number To Fractional String(number=w539, precision (6)=i16 1) -> (F-format string=w542:string)  [unwired: 2 in]
            n217 = Concatenate Strings(":" ("string"), "Kernel " ("string"), w560) -> (w538:string)
            n218 = Concatenate Strings(":" ("string"), "Kernel Size" ("string"), w557) -> (w537:string)
            n219 = Concatenate Strings(":" ("string"), "Filter Size X" ("string"), w554) -> (w536:string)
            n220 = Concatenate Strings(":" ("string"), "Filter Size Y" ("string"), w550) -> (w535:string)
            n221 = Concatenate Strings(":" ("string"), "Tolerance %" ("string"), w546) -> (w534:string)
            n222 = Concatenate Strings(":" ("string"), "Divider" ("string"), w542) -> (w533:string)
            n223 = Concatenate Strings(w538, w537, w536, w535, w534, w533) -> (w532:string)
          }
          frame "Convolution - Highlight Details" {
            n224 = Number To Decimal String(number=w592) -> (decimal integer string=w590:string)  [unwired: 1 in]
            n225 = Number To Decimal String(number=w585) -> (decimal integer string=w587:string)  [unwired: 1 in]
            n226 = Number To Decimal String(number=w581) -> (decimal integer string=w583:string)  [unwired: 1 in]
            n227 = Array To Spreadsheet String(array=w595, 3:"%f.1" ("format string")) -> (spreadsheet string=w593:string)  [unwired: 1 in]
            n228 = Number To Decimal String(number=w577) -> (decimal integer string=w579:string)  [unwired: 1 in]
            n229 = Number To Fractional String(number=w572, precision (6)=i16 1) -> (F-format string=w575:string)  [unwired: 2 in]
            n230 = Concatenate Strings(":" ("string"), "Kernel " ("string"), w593) -> (w571:string)
            n231 = Concatenate Strings(":" ("string"), "Kernel Size" ("string"), w590) -> (w570:string)
            n232 = Concatenate Strings(":" ("string"), "Filter Size X" ("string"), w587) -> (w569:string)
            n233 = Concatenate Strings(":" ("string"), "Filter Size Y" ("string"), w583) -> (w568:string)
            n234 = Concatenate Strings(":" ("string"), "Tolerance %" ("string"), w579) -> (w567:string)
            n235 = Concatenate Strings(":" ("string"), "Divider" ("string"), w575) -> (w566:string)
            n236 = Concatenate Strings(w571, w570, w569, w568, w567, w566) -> (w565:string)
          }
          frame "Convolution - Custom" {
            n237 = Number To Decimal String(number=w625) -> (decimal integer string=w623:string)  [unwired: 1 in]
            n238 = Number To Decimal String(number=w618) -> (decimal integer string=w620:string)  [unwired: 1 in]
            n239 = Number To Decimal String(number=w614) -> (decimal integer string=w616:string)  [unwired: 1 in]
            n240 = Array To Spreadsheet String(array=w628, 3:"%f.1" ("format string")) -> (spreadsheet string=w626:string)  [unwired: 1 in]
            n241 = Number To Decimal String(number=w610) -> (decimal integer string=w612:string)  [unwired: 1 in]
            n242 = Number To Fractional String(number=w605, precision (6)=i16 1) -> (F-format string=w608:string)  [unwired: 2 in]
            n243 = Concatenate Strings(":" ("string"), "Kernel " ("string"), w626) -> (w604:string)
            n244 = Concatenate Strings(":" ("string"), "Kernel Size" ("string"), w623) -> (w603:string)
            n245 = Concatenate Strings(":" ("string"), "Filter Size X" ("string"), w620) -> (w602:string)
            n246 = Concatenate Strings(":" ("string"), "Filter Size Y" ("string"), w616) -> (w601:string)
            n247 = Concatenate Strings(":" ("string"), "Tolerance %" ("string"), w612) -> (w600:string)
            n248 = Concatenate Strings(":" ("string"), "Divider" ("string"), w608) -> (w599:string)
            n249 = Concatenate Strings(w604, w603, w602, w601, w600, w599) -> (w598:string)
          }
        }
        n250 = Concatenate Strings(w97, w91) -> (w90:string)
        n251 = Build Array("Filters", w90) -> (w103:string[])
      }
      frame "Lookup Table" {
        n252 = Variant To Data(type="LookupTableParam", Variant=w640) -> (data=w638:T4)  [unwired: 1 in, 1 out]
        n253 = Unbundle By Name(w638) -> ("Function"=w633:T17, "Power Value"=w632:sgl)
        n254 = property on="Function" class="Enum (strict)"() -> ("Strings []"=w636:string[])  [unwired: 2 in, 2 out]
        n255 = Index Array(array=w636, index=w633) -> (element=w635:string)
        n256 = case shown="\"Power X\"" w633 {
          tunnel: w635 -> [w642 w649 w656 w663]
          tunnel: [w641 w643 w650 w657] -> w634
          tunnel: w632 -> [_ w648 w655 w662]
          frame "Equalizer", Default {
            n257 = Concatenate Strings(w642) -> (w641:string)
          }
          frame "Power X" {
            n258 = Number To Fractional String(number=w648, precision (6)=i16 1) -> (F-format string=w644:string)  [unwired: 2 in]
            n259 = Concatenate Strings(w649, ":" ("string"), "Power Value " ("string"), w644) -> (w643:string)
          }
          frame "Reverse" {
            n260 = Number To Fractional String(number=w655, precision (6)=i16 1) -> (F-format string=w651:string)  [unwired: 2 in]
            n261 = Concatenate Strings(w656, ":" ("string"), "Power Value " ("string"), w651) -> (w650:string)
          }
          frame "Power 1/X" {
            n262 = Number To Fractional String(number=w662, precision (6)=i16 1) -> (F-format string=w658:string)  [unwired: 2 in]
            n263 = Concatenate Strings(w663, ":" ("string"), "Power Value " ("string"), w658) -> (w657:string)
          }
        }
        n264 = Build Array("Lookup Table ", w634) -> (w631:string[])
      }
      frame "Particle Filter" {
        n265 = Variant To Data(type="ParticleFilterParam", Variant=w696) -> (data=w695:T2)  [unwired: 1 in, 1 out]
        n266 = Unbundle By Name(w695) -> ("Selection Values"=w691:T18, "Keep/Remove Particles (F)"=w686:bool, "Reject Border? (F)"=w679:bool, "Fill Holes? (F)"=w678:bool, "Connectivity 4/8 (8)"=w677:bool)
        n267 = for {
          tunnel: w691 -> [w726] mode=indexing
          shift-right: [w698] -> w689
          shift-left: "" -> [w700]
          n268 = Unbundle By Name(w726) -> ("Measurement Parameter"=w724:T3, "Range Lower Value"=w720:dbl, "Range Upper Value"=w716:dbl, "Range"=w709:bool, "Measurement Type"=w703:bool)
          n269 = property on="Measurement Parameter" class="Ring (strict)"() -> ("Strings []"=w725:string[])  [unwired: 2 in, 2 out]
          n270 = Index Array(array=w725, index=w724) -> (element=w723:string)
          n271 = Number To Fractional String(number=w720, precision (6)=i16 2) -> (F-format string=w718:string)  [unwired: 2 in]
          n272 = Number To Fractional String(number=w716, precision (6)=i16 2) -> (F-format string=w713:string)  [unwired: 2 in]
          n273 = Select(t="True" ("delimiter (Tab)"), s=w703, f="False" ("delimiter (Tab)")) -> (s? t:f=w701:string)
          n274 = Select(t="True" ("delimiter (Tab)"), s=w709, f="False" ("delimiter (Tab)")) -> (s? t:f=w707:string)
          n275 = Concatenate Strings(w723, ":" ("string"), "Range Lower Value " ("string"), w718, ":" ("string"), "Range Upper Value" ("string"), w713, ":" ("string"), "Range" ("string"), w707, ":" ("string"), "Measurement Type " ("string"), w701, ":" ("string")) -> (w699:string)
          n276 = Concatenate Strings(w700, w699) -> (w698:string)
        }
        n277 = Select(t="True" ("delimiter (Tab)"), s=w677, f="False" ("delimiter (Tab)")) -> (s? t:f=w665:string)
        n278 = Select(t="True" ("delimiter (Tab)"), s=w686, f="False" ("delimiter (Tab)")) -> (s? t:f=w675:string)
        n279 = Select(t="True" ("delimiter (Tab)"), s=w679, f="False" ("delimiter (Tab)")) -> (s? t:f=w673:string)
        n280 = Select(t="True" ("delimiter (Tab)"), s=w678, f="False" ("delimiter (Tab)")) -> (s? t:f=w670:string)
        n281 = Concatenate Strings(w689, ":" ("string"), "Keep/Remove" ("string"), w675, ":" ("string"), "Reject Border " ("string"), w673, ":" ("string"), "Fill Hole " ("string"), w670, ":" ("string"), "Connectivity 4/8 " ("string"), w665) -> (w664:string)
        n282 = Build Array("Particle Filter ", w664) -> (w693:string[])
      }
      frame "None", Default {
      }
    }
    n283 = Equal?(x=w9, y=string[] ["", ""]) -> (x = y?=w8:bool[])
    n284 = And Array Elements(Boolean array=w8) -> (logical AND=w7:bool)
    n285 = Not(x=w7) -> (.not. x?=w5:bool)
  }
  n286 = property class="MCListbox (strict)"(reference="ProcessSteps", "ItemNames"=w2) -> ()  [unwired: 1 in, 2 out]
  "error out" <- "error in (no error)"
